vi "Thermal_type.vi"() -> ()   [LabVIEW 2016]
panel:
  in  "small scan range?":bool
  out "SysPulserSelA":i16
  in  "Min.Depth":bool
  in  "Max.PRF":bool
  in  "Measurement Type":enum32{"Volt", "SA"}(radio)
  in  "System \nSelection":enum32{"Common", "Frosk", "Griffin", "K2"}(radio)
  out "Type Transducer":string="Phase"
  in  "Target temperature data":dbl[](array[numeric])=[35.0, 35.0, 35.0, 35.0, 35.0, 35.0, 35.0, 35.0, 35.0, 35.0]
  in  "Measured time for SA":enum32{"5min", "30min"}(radio)
  in  "Selection system":bool
  in  "Measured time for volt":enum32{"5min", "30min"}(radio)
  in  "PID(search PRF)":bool=TRUE
  in  "Initial PRF":dbl format="%.2f"
  in  "measSetId(For SA)":string="29, 37, 44"
  out "meaSetId(Volt)":i32[](array[numeric])
  out "meaSetId(SA)":i32[](array[numeric])
  out "Large RoiMin":dbl
  out "Large RoiSpan":dbl
  out "Small TxElement":i32
  out "Monitoring PRF":dbl
  out "Roi Lat Span":dbl format="%.2f"
  out "Roi Lat Min":dbl format="%.2f"
  in  "VISA resource name":refnum<visa-resource-name>="COM1"
  in  "Thermometer Type":u16(ring) items=["HH506R", "HH506RA"]
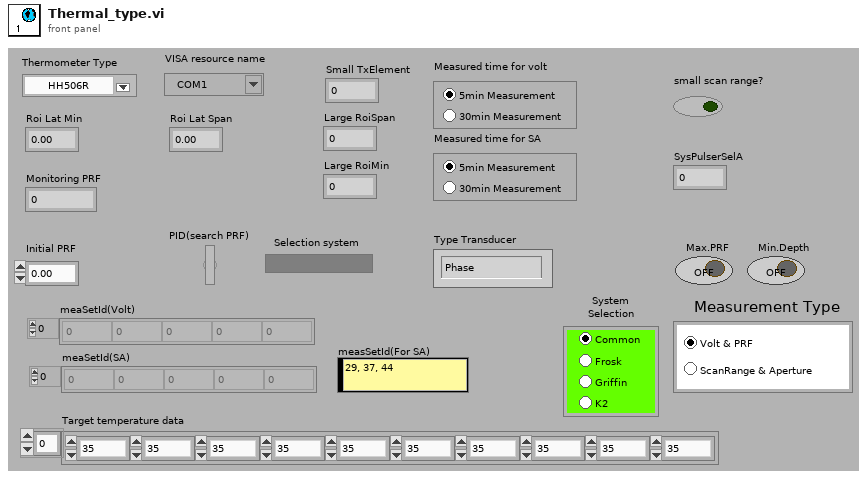
[diagram p1: front panel]
diagram:
